vi "Scan Read Formatted.vi"(8 "error in (no error)":errorcluster {"code" format="%.0x"}, 9 "ValBufferSize":i32=256, 10 "MaxTimeMilliseconds":i32 format="%.0g", 11 "instrument handle":refnum<k15>) -> (0 "error out":errorcluster {"code" format="%.0x"}, 2 "Val":string, 3 "instrument handle out":refnum<k15>)   [LabVIEW 2020, in "Keysight DAQ970.lvlib"]
doc: "Change the state of the triggering system from the 'idle' state to the 'wait-for-trigger' state. Scanning of the current list will begin once the specified trigger conditions are satisfied. Readings are sent immediately to the instrument's output buffer."
uses:
  Keysight DAQ970.lvlib
  KtDAQ970.dll
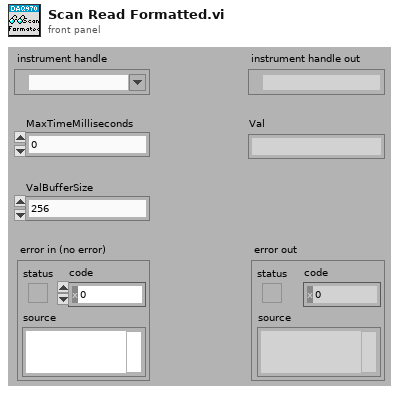
[diagram p1: front panel]
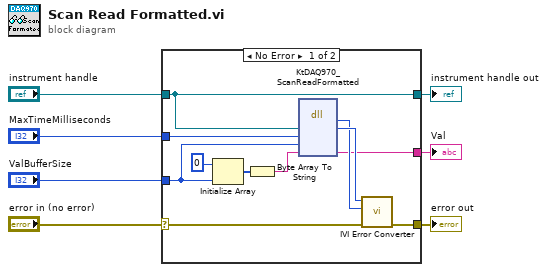
[diagram p0: block diagram]
diagram:
  n1 = case shown="No Error" "error in (no error)" {
    selector: "error in (no error)" -> [w16 w20]
    tunnel: [w15 w20] -> w7
    tunnel: "instrument handle" -> [w10 w19]
    tunnel: "MaxTimeMilliseconds" -> [w14 _]
    tunnel: "ValBufferSize" -> [w9 _]
    tunnel: [w11 _] -> w2
    tunnel: [w10 w19] -> w1
    frame No Error {
      n2 = Initialize Array(u8 0 ("element"), w9) -> (w13:u8[])
      n3 = Byte Array To String(unsigned byte array=w13) -> (string=w8:string)
      n4 = dll-call lib="KtDAQ970**.dll" fn="KtDAQ970_ScanReadFormatted"("Vi"=w10, "MaxTimeMilliseconds"=w14, "ValBufferSize"=w9, "Val"=w8) -> (w17:i32, "Vi"=w18:u32, "Val"=w11:string)  [unwired: 5 in, 2 out]
      n5 = call "IVI Error Converter.vi"("error in (no error)"=w16, "IVI error code (0)"=w17, "instrument handle"=w18) -> ("error out"=w15:errorcluster)  [unwired: 7 in, 1 out]
    }
    frame Error {
    }
  }
  "error out" <- w7
  "instrument handle out" <- w1
  "Val" <- w2
